vi "Add Points to Series_DBL[].vi"(6 "YValuesPerPoint":i32=1, 8 "error in (no error)":errorcluster, 9 "Data":cluster{"X":dbl, "Y":dbl}[](array[cluster])=[{"X"=0.0, "Y"=0.25}, {"X"=1.0, "Y"=0.75}, {"X"=2.0, "Y"=1.95}, {"X"=3.0, "Y"=1.6}, {"X"=4.0, "Y"=1.6}, {"X"=5.0, "Y"=2.5}, {"X"=6.0, "Y"=1.8}, {"X"=7.0, "Y"=1.26}], 10 ".NET MSChart Series":refnum<k24>) -> (0 "error out":errorcluster, 2 ".NET MSChart Series (dup)":refnum<k24>)   [LabVIEW 2014, in "XMSChart.xctl"]
uses:
  XMSChart.xctl
  System.Windows.Forms.DataVisualization
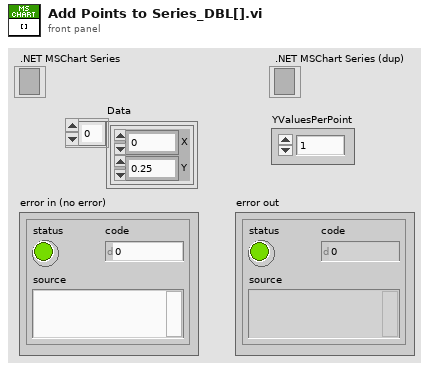
[diagram p1: front panel]
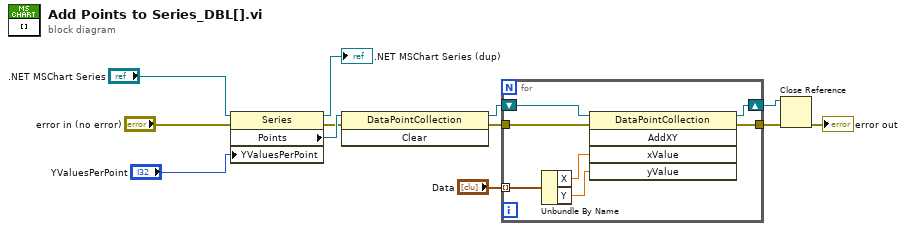
[diagram p0: block diagram]
diagram:
  n1 = property on="Property Node" class="Series"(reference=".NET MSChart Series", error in="error in (no error)", "YValuesPerPoint"="YValuesPerPoint") -> (reference out=→".NET MSChart Series (dup)":refnum<k24>, error out=w2:errorcluster, "Points"=w9:refnum<k24>)
  n2 = invoke on="Invoke Node" class="DataPointCollection" method="Clear"(reference=w9, error in=w2) -> (reference out=w3:refnum<k24>, error out=w1:errorcluster)  [unwired: 1 in, 1 out]
  n3 = for {
    tunnel: "Data" -> [w14] mode=indexing
    tunnel: [w17] -> w6
    shift-right: [w18] -> w7
    shift-left: w3 -> [w19]
    tunnel: w1 -> [w16]
    n4 = Unbundle By Name(w14) -> ("X"=w13:dbl, "Y"=w15:dbl)
    n5 = invoke class="DataPointCollection" method="AddXY"(reference=w19, error in=w16, "xValue"=w13, "yValue"=w15) -> (reference out=w18:refnum<k24>, error out=w17:errorcluster)  [unwired: 1 in, 3 out]
  }
  n6 = Close Reference(reference=w7, error in (no error)=w6) -> (error out=→"error out":errorcluster)
